vi "process.vi"(8 "error in (no error)":errorcluster, 9 "Calling VI Reference i":refnum<vi>, 10 "GObj Refnum":refnum<vi>, 11 "MultiFrameStructure in":refnum<class "MultiFrameStructure.lvclass">) -> (0 "error out":errorcluster, 3 "MultiFrameStructure out":refnum<class "MultiFrameStructure.lvclass">)   [LabVIEW 2016, in "MultiFrameStructure.lvclass"]
uses:
  MultiFrameStructure.lvclass
  C:/LSST_TS/SystemSW/ct_tools/GObject/GObject.lvclass
  Dependency/Dependency.lvclass
  DiagramObject/DiagramObject.lvclass
  GObject/GObject.lvclass/GObject.ctl
  DiagramObject/DiagramObject.lvclass/DiagramObject.ctl
  Dependency/Dependency.lvclass/Dependency.ctl
  GObject/GObject.lvclass
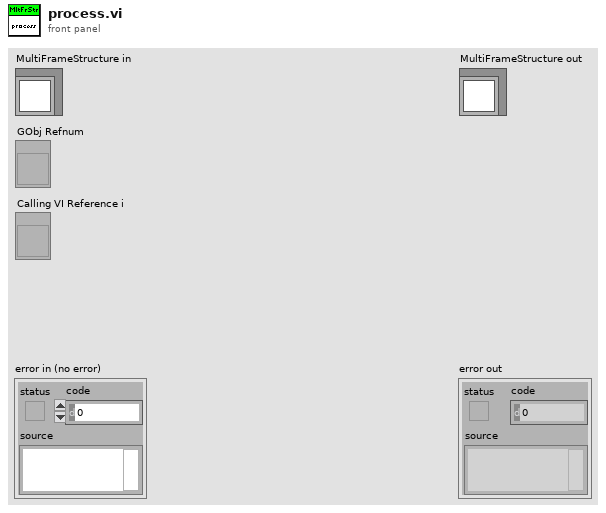
[diagram p1: front panel]
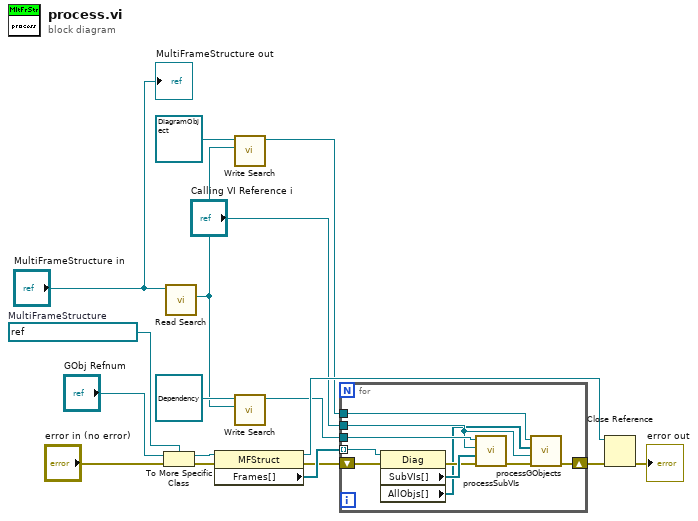
[diagram p0: block diagram]
diagram:
  w14 = refnum<vi> refnum  # MultiFrameStructure
  n1 = To More Specific Class(target class=w14, reference="GObj Refnum", error in="error in (no error)") -> (specific class reference=w17:refnum<vi>, error out=w16:errorcluster)
  n2 = call "Read Search.vi"("DiagramObject in"="MultiFrameStructure in") -> ("Search.lvclass"=w5:refnum<class "Search.lvclass">)  [unwired: 9 in, 1 out]
  n3 = property class="MFStruct"(reference=w17, error in=w16) -> (reference out=w12:refnum<vi>, error out=w1:errorcluster, "Frames[]"=w15:refnum<vi>[])
  n4 = call "Write Search.vi"("Search"=w5, "DiagramObject in"=refnum<class "DiagramObject.lvclass"> refnum ("DiagramObject.lvclass")) -> ("DiagramObject out"=w4:refnum<class "DiagramObject.lvclass">)  [unwired: 9 in]
  n5 = call "Write Search.vi"("Search"=w5, "Dependency in"=refnum<class "Dependency.lvclass"> refnum ("Dependency.lvclass")) -> ("Dependency out"=w10:refnum<class "Dependency.lvclass">)  [unwired: 9 in]
  n6 = for {
    tunnel: w15 -> [w27] mode=indexing
    tunnel: "Calling VI Reference i" -> [w21]
    shift-right: [w18] -> w13
    shift-left: w1 -> [w26]
    tunnel: w10 -> [w25]
    tunnel: w4 -> [w19]
    n7 = property class="Diag"(reference=w27, error in=w26) -> (error out=w23:errorcluster, "SubVIs[]"=w24:refnum<vi>[], "AllObjs[]"=w20:refnum<vi>[])  [unwired: 1 out]
    n8 = call "processSubVIs.vi"("error in (no error)"=w23, "SubVIs[]"=w24, "Calling VI Reference i"=w21, "Dependency in"=w25) -> ("error out"=w22:errorcluster)  [unwired: 5 in, 2 out]
    n9 = call "processGObjects.vi"("error in (no error)"=w22, "Calling VI Reference i"=w21, "All Objects[]"=w20, "DiagramObject in"=w19) -> ("error out"=w18:errorcluster)  [unwired: 6 in, 1 out]
  }
  n10 = Close Reference(reference=w12, error in (no error)=w13) -> (error out=→"error out":errorcluster)
  "MultiFrameStructure out" <- "MultiFrameStructure in"
